vi "turn.vi"(8 "angle (ccw)":dbl, 9 "speed (%)":dbl, 10 "rightMotor":T1={"DeviceStatus"={"status"=FALSE, "code"=0, "source"=""}, "Type"=enum."PWM", "PWM"={"PWM Channel"=enum."Invalid", "DeadBand"={"Name"="", "maxPositivePwm"=0, "minPositivePwm"=0, "centerPwm"=0, "maxNegativePwm"=0, "minNegativePwm"=0, "angularRange"=0}}, "CAN"={"Device Number"=0, "SetOutput VI Ref"=variant(refnum<vi> refnum), "GetOutput VI Ref"=variant(refnum<vi> refnum), "Enable VI Ref"=variant(refnum<vi> refnum), "Disable VI Ref"=variant(refnum<vi> refnum), "Data"=variant}, "Invert"=FALSE}, 11 "leftMotor":T1={"DeviceStatus"={"status"=FALSE, "code"=0, "source"=""}, "Type"=enum."PWM", "PWM"={"PWM Channel"=enum."Invalid", "DeadBand"={"Name"="", "maxPositivePwm"=0, "minPositivePwm"=0, "centerPwm"=0, "maxNegativePwm"=0, "minNegativePwm"=0, "angularRange"=0}}, "CAN"={"Device Number"=0, "SetOutput VI Ref"=variant(refnum<vi> refnum), "GetOutput VI Ref"=variant(refnum<vi> refnum), "Enable VI Ref"=variant(refnum<vi> refnum), "Disable VI Ref"=variant(refnum<vi> refnum), "Data"=variant}, "Invert"=FALSE}) -> (2 "rightMotor":T1={"DeviceStatus"={"status"=FALSE, "code"=0, "source"=""}, "Type"=enum."PWM", "PWM"={"PWM Channel"=enum."Invalid", "DeadBand"={"Name"="", "maxPositivePwm"=0, "minPositivePwm"=0, "centerPwm"=0, "maxNegativePwm"=0, "minNegativePwm"=0, "angularRange"=0}}, "CAN"={"Device Number"=0, "SetOutput VI Ref"=variant(enum8{"Percent VBus", "Current", "Speed", "Position", "Voltage"} enum."Percent VBus"), "GetOutput VI Ref"=variant(refnum<k1> refnum), "Enable VI Ref"=variant(dbl 12.0), "Disable VI Ref"=variant(enum8{"Percent VBus", "Speed", "Position", "Slave", "Unchanged / Invalid"} enum."Percent VBus"), "Data"=variant}, "Invert"=FALSE}, 3 "leftMotor":T1={"DeviceStatus"={"status"=FALSE, "code"=0, "source"=""}, "Type"=enum."PWM", "PWM"={"PWM Channel"=enum."Invalid", "DeadBand"={"Name"="", "maxPositivePwm"=0, "minPositivePwm"=0, "centerPwm"=0, "maxNegativePwm"=0, "minNegativePwm"=0, "angularRange"=0}}, "CAN"={"Device Number"=0, "SetOutput VI Ref"=variant(enum8{"Percent VBus", "Current", "Speed", "Position", "Voltage"} enum."Percent VBus"), "GetOutput VI Ref"=variant(refnum<k1> refnum), "Enable VI Ref"=variant(dbl 12.0), "Disable VI Ref"=variant(enum8{"Percent VBus", "Speed", "Position", "Slave", "Unchanged / Invalid"} enum."Percent VBus"), "Data"=variant}, "Invert"=FALSE})   [LabVIEW 2016]
uses:
  <vilib>/Rock Robotics/WPI/MotorControl/WPI_MotorControlDeviceRef.ctl
  <vilib>/Rock Robotics/WPI/MotorControl/WPI_MotorControlType.ctl
  <vilib>/Rock Robotics/SystemInterfaces/DIO/FPGA_DIOPWMChannel.ctl
  <vilib>/Rock Robotics/WPI/PWM/WPI_PWMDeadband.ctl
  <vilib>/Rock Robotics/WPI/ThirdParty/Sensors/navX/_TypeDefs/FRIC_navX_DeviceNumbersTypeDef.ctl
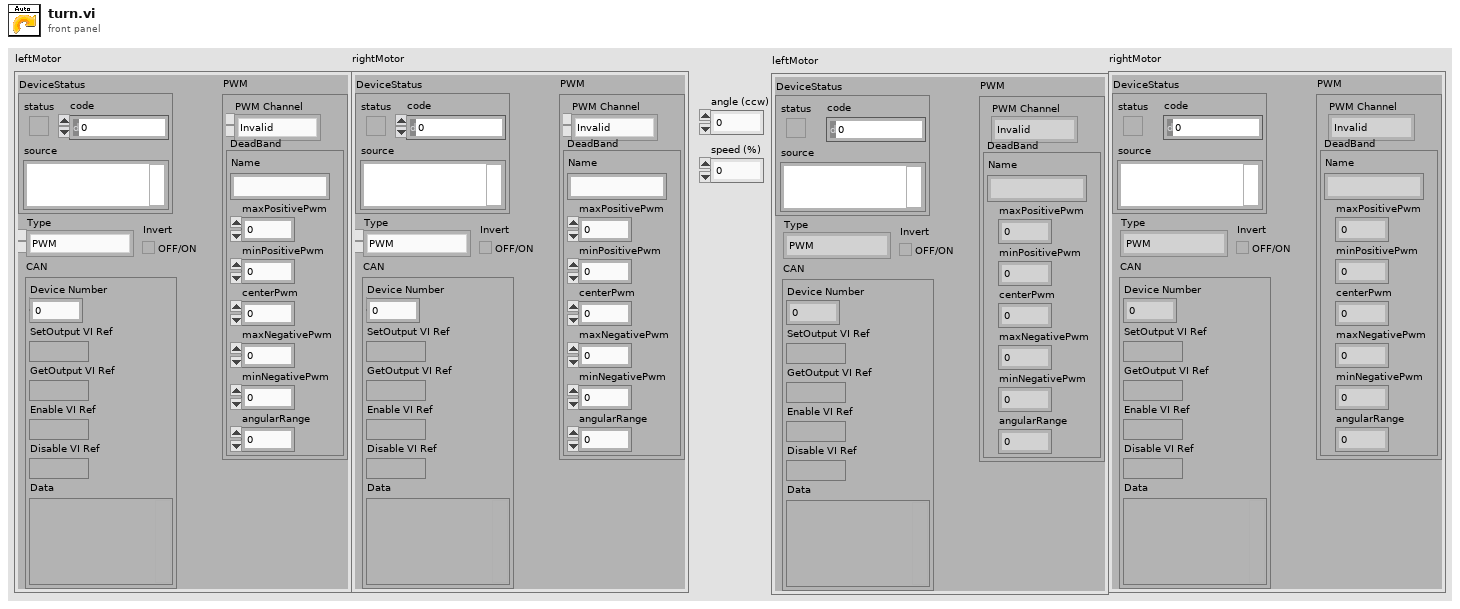
[diagram p1: front panel]
types:
  T1 = typedef "WPI_MotorControlDeviceRef.ctl" = cluster{"DeviceStatus":errorcluster, "Type":T2, "PWM":cluster{"PWM Channel":T3, "DeadBand":T4}, "CAN":cluster{"Device Number":u8, "SetOutput VI Ref":variant, "GetOutput VI Ref":variant, "Enable VI Ref":variant, "Disable VI Ref":variant, "Data":variant}, "Invert":bool}
  T2 = typedef "WPI_MotorControlType.ctl" = enum16{"PWM", "CAN"}
  T3 = typedef "FPGA_DIOPWMChannel.ctl" = enum8{"PWM 0", "PWM 1", "PWM 2", "PWM 3", "PWM 4", "PWM 5", "PWM 6", "PWM 7", "PWM 8", "PWM 9", "PWM MXP 0", "PWM MXP 1", "PWM MXP 2", "PWM MXP 3", "PWM MXP 4", "PWM MXP 5", "PWM MXP 6", "PWM MXP 7", "PWM MXP 8", "PWM MXP 9", "Invalid"}
  T4 = typedef "WPI_PWMDeadband.ctl" = cluster{"Name":string, "maxPositivePwm":i32, "minPositivePwm":i32, "centerPwm":i32, "maxNegativePwm":i32, "minNegativePwm":i32, "angularRange":u16}
  T5 = typedef "FRIC_navX_DeviceNumbersTypeDef.ctl" = enum16{"Dev0", "Dev1", "Dev2", "Dev3"}
  T6 = cluster{"Yaw":dbl, "Roll":dbl, "Pitch":dbl, "Heading":dbl, "Fused Heading":dbl}
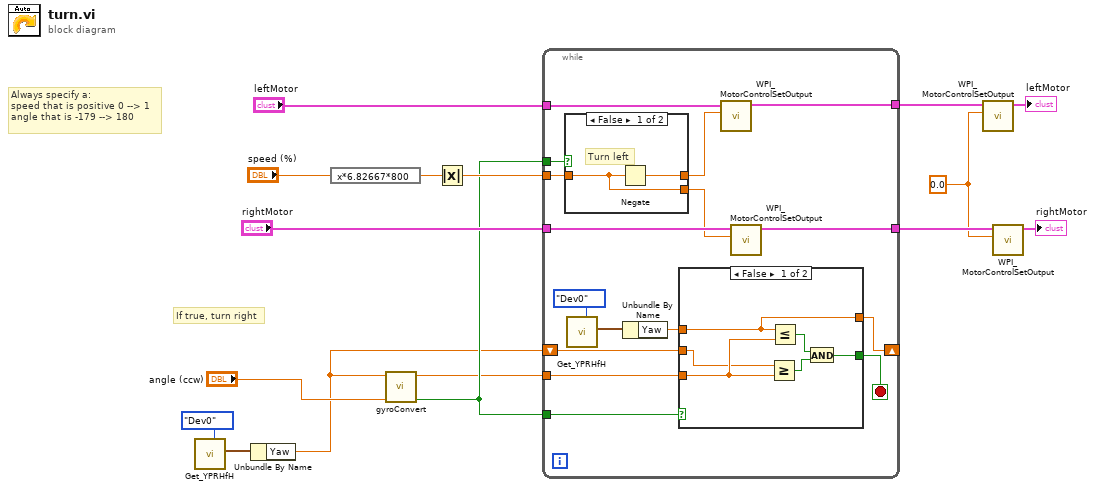
[diagram p0: block diagram]
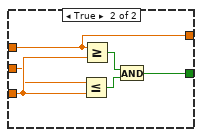
[diagram p2: hidden frame]
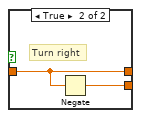
[diagram p3: hidden frame]
diagram:
  w9 = 0.0
  # "Always specify a:\nspeed that is positive 0 --> 1\nangle that is -179 --> 180"
  # "If true, turn right"
  n1 = call <vilib>:"Get_YPRHfH.vi"("Device Number"=FRIC_navX_DeviceNumbersTypeDef."Dev0") -> ("YRPHfH"=w1:T6)  [unwired: 10 in]
  n2 = Unbundle By Name(w1) -> ("Yaw"=w3:dbl)
  n3 = expression code="x*6.82667*800"("speed (%)") -> (w13:dbl)
  n4 = call "gyroConvert.vi"("turnThis (-180 to 180)"="angle (ccw)", "angle (-180 to 180)"=w3) -> ("turnRight"=w5:bool, "neededAngle (-180 to 180)"=w4:dbl)  [unwired: 8 in]
  n5 = Absolute Value(x=w13) -> (abs(x)=w12:dbl)
  n6 = while {
    tunnel: "leftMotor" -> [w30]
    tunnel: "rightMotor" -> [w29]
    tunnel: w12 -> [w28]
    tunnel: [w25] -> w11
    tunnel: [w24] -> w10
    tunnel: w5 -> [w23]
    tunnel: w5 -> [w22]
    tunnel: w4 -> [w20]
    shift-right: [w19] -> _
    shift-left: w3 -> [w18]
    stop <- w21 stop-if-true
    n7 = case shown="False" w23 {
      tunnel: w28 -> [w45 w48]
      tunnel: [w46 w48] -> w27
      tunnel: [w45 w47] -> w26
      frame False {
        # "Turn left"
        n8 = Negate(x=w45) -> (-x=w46:dbl)
      }
      frame True {
        # "Turn right"
        n9 = Negate(x=w48) -> (-x=w47:dbl)
      }
    }
    n10 = call <vilib>:"Get_YPRHfH.vi"("Device Number"=FRIC_navX_DeviceNumbersTypeDef."Dev0") -> ("YRPHfH"=w31:T6)  [unwired: 10 in]
    n11 = Unbundle By Name(w31) -> ("Yaw"=w17:dbl)
    n12 = case shown="False" w22 {
      tunnel: [w38 w44] -> w21
      tunnel: w20 -> [w35 w41]
      tunnel: w17 -> [w34 w39]
      tunnel: [w34 w39] -> w19
      tunnel: w18 -> [w33 w40]
      frame False {
        n13 = Greater Or Equal?(x=w33, y=w35) -> (x >= y?=w37:bool)
        n14 = Less Or Equal?(x=w34, y=w35) -> (x <= y?=w36:bool)
        n15 = And(x=w36, y=w37) -> (x .and. y?=w38:bool)
      }
      frame True {
        n16 = Less Or Equal?(x=w40, y=w41) -> (x <= y?=w42:bool)
        n17 = Greater Or Equal?(x=w39, y=w41) -> (x >= y?=w43:bool)
        n18 = And(x=w43, y=w42) -> (x .and. y?=w44:bool)
      }
    }
    n19 = call <vilib>:"WPI_MotorControlSetOutput.vi"("Output"=w27, "MotorControlDevRef"=w30) -> ("MotorControlDevRef"=w25:T1)  [unwired: 7 in, 2 out]
    n20 = call <vilib>:"WPI_MotorControlSetOutput.vi"("Output"=w26, "MotorControlDevRef"=w29) -> ("MotorControlDevRef"=w24:T1)  [unwired: 7 in, 2 out]
  }
  n21 = call <vilib>:"WPI_MotorControlSetOutput.vi"("Output"=w9, "MotorControlDevRef"=w11) -> ("MotorControlDevRef"=→"leftMotor":T1)  [unwired: 7 in, 2 out]
  n22 = call <vilib>:"WPI_MotorControlSetOutput.vi"("Output"=w9, "MotorControlDevRef"=w10) -> ("MotorControlDevRef"=→"rightMotor":T1)  [unwired: 7 in, 2 out]
